vi "Easy_Test1.vi"() -> ()   [LabVIEW 2014]
panel:
  out "String Out":string
  in  "String In":string
  # "Convert a string of hex ASCII values to an ASCII string"
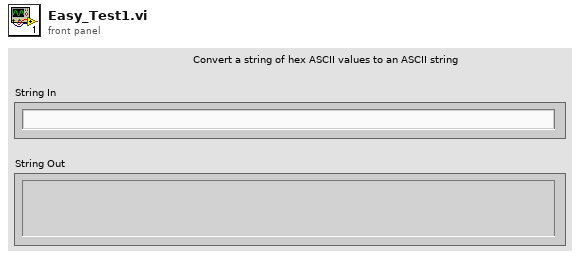
[diagram p1: front panel]
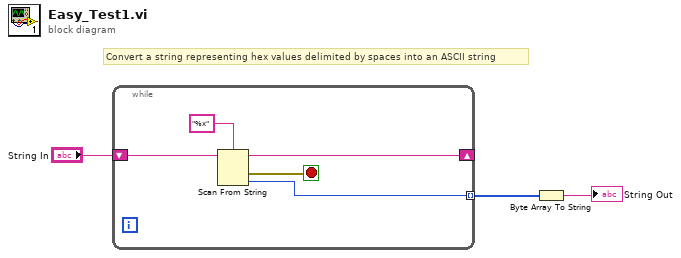
[diagram p0: block diagram]
diagram:
  # "Convert a string representing hex values delimited by spaces into an ASCII string"
  n1 = while {
    shift-right: [w6] -> _
    shift-left: "String In" -> [w7]
    tunnel: [w5] -> w2 mode=indexing
    stop <- w4 stop-if-true
    n2 = Scan From String "Scan From String"(format string="%x", input string=w7) -> (remaining string=w6:string, error out=w4:errorcluster, output 1=w5:u32)  [unwired: 3 in, 1 out]
  }
  n3 = Byte Array To String(unsigned byte array=w2) -> (string=→"String Out":string)
